vi "svl_Check Data Valid [Level] [Resampled] (N Ch).vi"(0 "scaled even angle signals [EU]":T5(array[cluster]) {"even angle signal" format="%.2f"; "dr" format="%.2f"; "r0" format="%.2f"}, 1 "exponential mode":enum16{"Slow", "Fast", "Impulse", "Custom"}(ring)=enum."Fast", 2 "time constant [ms]":dbl=125.0 format="%.2f", 5 "even angle channel info":T1[](array[typedef]) {"channel info"."pregain" format="%.2f"; "channel info"."weighting filter" items=["Linear", "A-weighting", "B-weighting", "C-weighting", "ITU-R 468-4", "Dolby", "CCITT", "C-message", "Wb", "Wc", "Wd", "We", "Wf", "Wh", "Wj", "Wk", "Wm", "AES17 20 kHz lowpass", "AES17 40 kHz lowpass", "AES17 20 kHz highpass", "AES17 40 kHz highpass"]; "channel info"."dB reference" format="%^.1e"; "channel info"."engineering units" items=["custom..."=0, "V"=1, "A"=21, "C"=30, "pC"=31, "s"=32, "-"=29, "Pa"=2, "N"=20, "g"=3, "m/s^2"=4, "m/s"=5, "m"=6, "mm/s"=12, "mm"=13, "micron/s"=14, "micron"=15, "in/s^2"=7, "in/s"=8, "in"=9, "mil/s"=10, "mil"=11, "rad/s^2"=16, "rad/s"=17, "rad"=18, "deg/s^2"=26, "deg/s"=27, "deg"=28, "RPM"=22, "cycle/s^2"=23, "Hz"=24, "cycle"=25, "strain"=19]; "channel info"."sensor sensitivity" format="%#_5f"}, 7 "level analysis":T7(ring), 9 "restart averaging (F)":bool, 11 "error in (no error)":errorcluster, 12 "integration time [s]":dbl=1.0 format="%.2f", 13 "decimation factor":i32=1 min=1 step=1) -> (4 "dup scaled even angle signals [EU]":T5(array[cluster]) {"even angle signal" format="%.2f"; "dr" format="%.2f"; "r0" format="%.2f"}, 6 "dup even angle channel info":T1[](array[typedef]) {"channel info"."pregain" format="%.2f"; "channel info"."weighting filter" items=["Linear", "A-weighting", "B-weighting", "C-weighting", "ITU-R 468-4", "Dolby", "CCITT", "C-message", "Wb", "Wc", "Wd", "We", "Wf", "Wh", "Wj", "Wk", "Wm", "AES17 20 kHz lowpass", "AES17 40 kHz lowpass", "AES17 20 kHz highpass", "AES17 40 kHz highpass"]; "channel info"."dB reference" format="%^.1e"; "channel info"."engineering units" items=["custom..."=0, "V"=1, "A"=21, "C"=30, "pC"=31, "s"=32, "-"=29, "Pa"=2, "N"=20, "g"=3, "m/s^2"=4, "m/s"=5, "m"=6, "mm/s"=12, "mm"=13, "micron/s"=14, "micron"=15, "in/s^2"=7, "in/s"=8, "in"=9, "mil/s"=10, "mil"=11, "rad/s^2"=16, "rad/s"=17, "rad"=18, "deg/s^2"=26, "deg/s"=27, "deg"=28, "RPM"=22, "cycle/s^2"=23, "Hz"=24, "cycle"=25, "strain"=19]; "channel info"."sensor sensitivity" format="%#_5f"}, 10 "processing state":T6(ring), 15 "error out":errorcluster)   [LabVIEW 2017]
uses:
  <vilib>/addons/_NISVFA/_Shared subVIs/Controls/svc_Resampled Channel Info.ctl
  <vilib>/addons/_NISVFA/_Shared subVIs/Controls/svc_Channel Info.ctl
  <vilib>/addons/_NISVFA/_Shared subVIs/Controls/svc_Engineering Units Text Ring.ctl
  <vilib>/addons/_NISVFA/_Shared subVIs/Controls/svc_Weighting Filter Text Ring.ctl
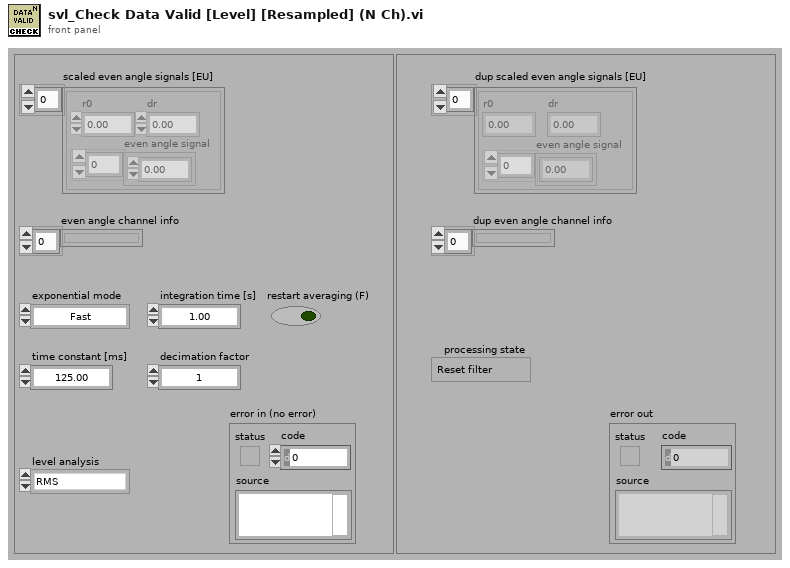
[diagram p1: front panel]
types:
  T1 = typedef "svc_Resampled Channel Info.ctl" = cluster{"channel name":string, "description":string, " channel info":T2}
  T2 = typedef "svc_Channel Info.ctl" = cluster{"sensor sensitivity":dbl, "engineering units":T3, "dB reference":dbl, "custom label":string, "weighting filter":T4, "pregain":dbl}
  T3 = typedef "svc_Engineering Units Text Ring.ctl" = u16
  T4 = typedef "svc_Weighting Filter Text Ring.ctl" = u16
  T5 = cluster{"r0":dbl, "dr":dbl, "even angle signal":dbl[]}[]
  T6 = enum16{"Reset filter", "Restart averaging", "Continue processing"}
  T7 = enum16{"RMS", "Running RMS", "Exp avg  ", "Dec exp avg ", "Peak", "Crest"}
  T8 = cluster{"ignore dt's equal":bool, "ignore array lengths equal":bool, "ignore # channels":bool}
  T9 = cluster{"ignore dt":bool, "ignore t0 continuity":bool, "ignore array length":bool, "ignore channel info":bool, "ignore channel name":bool}
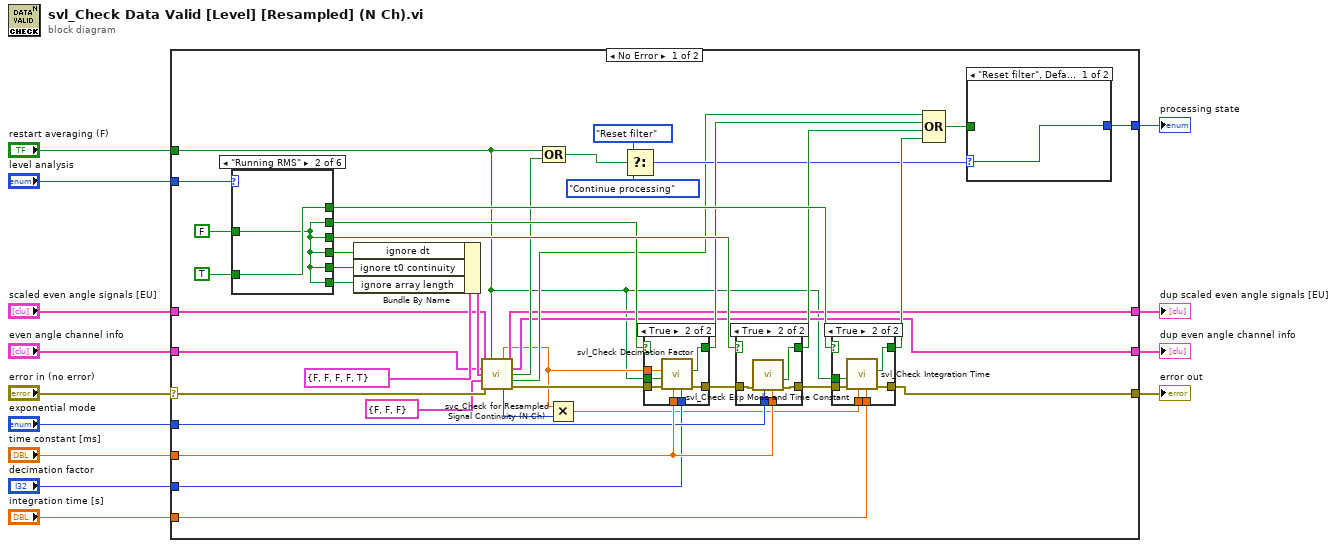
[diagram p0: block diagram]
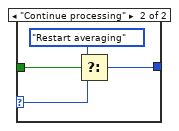
[diagram p10: hidden frame]
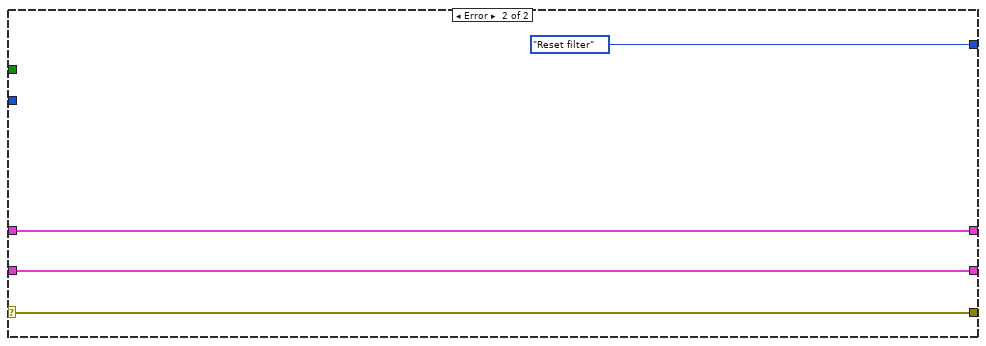
[diagram p11: hidden frame]
diagram:
  n1 = case shown="No Error" "error in (no error)" {
    selector: "error in (no error)" -> [w27 w98]
    tunnel: [w26 w98] -> w12
    tunnel: "scaled even angle signals [EU]" -> [w32 w96]
    tunnel: "restart averaging (F)" -> [w14 _]
    tunnel: "time constant [ms]" -> [w31 _]
    tunnel: [w53 T6."Reset filter" ("processing state")] -> w9
    tunnel: "level analysis" -> [w33 _]
    tunnel: "integration time [s]" -> [w28 _]
    tunnel: "decimation factor" -> [w29 _]
    tunnel: "exponential mode" -> [w30 _]
    tunnel: [w20 w96] -> w3
    tunnel: "even angle channel info" -> [w19 w95]
    tunnel: [w18 w95] -> w1
    frame No Error {
      n2 = case shown="\"Running RMS\"" w33 {
        tunnel: [w79 w80 w82 w84 w87 w89] -> w49
        tunnel: [w79 w80 w83 w84 w87 w89] -> w48
        tunnel: [w79 w81 w83 w85 w87 w89] -> w47
        tunnel: [w78 w80 w82 w84 w86 w88] -> w34
        tunnel: [w78 w80 w83 w85 w86 w88] -> w43
        tunnel: [w79 w80 w83 w85 w86 w89] -> w42
        tunnel: FALSE -> [w79 w80 w83 w85 w87 w89]
        tunnel: TRUE -> [w78 w81 w82 w84 w86 w88]
        frame "RMS", Default {
        }
        frame "Running RMS" {
        }
        frame "Exp avg  " {
        }
        frame "Dec exp avg " {
        }
        frame "Peak" {
        }
        frame "Crest" {
        }
      }
      n3 = Bundle By Name(cluster=T9 {"ignore dt"=FALSE, "ignore t0 continuity"=FALSE, "ignore array length"=FALSE, "ignore channel info"=FALSE, "ignore channel name"=TRUE} ("parameter controls"), "ignore dt"=w42, "ignore t0 continuity"=w43, "ignore array length"=w34) -> (w44:T9)
      n4 = call <vilib>:"svc_Check for Resampled Signal Continuity (N Ch).vi"("even angle signals"=w32, "restart averaging (F)"=w14, "even angle channel info"=w19, "parameter controls"=w44, "multichannel parameter controls"=T8 {"ignore dt's equal"=FALSE, "ignore array lengths equal"=FALSE, "ignore # channels"=FALSE}, "error in (no error)"=w27) -> ("dr"=w17:dbl, "dup even angle signals"=w20:T5, "dup even angle channel info"=w18:T1[], "waveform parameter changed"=w22:bool, "multichannel parameter changed"=w21:bool, "array length"=w16:i32, "error out"=w39:errorcluster)  [unwired: 3 in]
      n5 = Compound Arithmetic op=OR(w14, w22) -> (w46:bool)
      n6 = Multiply(x=w17, y=w16) -> (x*y=w15:dbl)
      n7 = Select(t=T6."Reset filter" ("processing state"), s=w46, f=T6."Continue processing" ("processing state")) -> (s? t:f=w25:T6)
      n8 = case shown="True" w48 {
        selector: w48 -> [w62 _]
        tunnel: w39 -> [w63 w70]
        tunnel: [w63 w69] -> w41
        tunnel: w31 -> [_ w68]
        tunnel: w29 -> [_ w67]
        tunnel: [w62 w65] -> w37
        tunnel: w17 -> [_ w66]
        tunnel: w14 -> [_ w64]
        frame False {
        }
        frame True {
          n9 = call <vilib>:"svl_Check Decimation Factor.vi"("decimation factor"=w67, "time constant [ms]"=w68, "error in (no error)"=w70, "restart averaging (F)"=w64, "dt"=w66) -> ("error out"=w69:errorcluster, "parameter has changed"=w65:bool)  [unwired: 5 in]
        }
      }
      n10 = case shown="True" w49 {
        selector: w49 -> [w71 _]
        tunnel: w30 -> [_ w77]
        tunnel: w41 -> [w72 w73]
        tunnel: [w72 w76] -> w40
        tunnel: [w71 w74] -> w38
        tunnel: w31 -> [_ w75]
        frame False {
        }
        frame True {
          n11 = call <vilib>:"svl_Check Exp Mode and Time Constant.vi"("time constant [ms]"=w75, "exponential mode"=w77, "error in (no error)"=w73) -> ("error out"=w76:errorcluster, "parameter has changed"=w74:bool)  [unwired: 7 in]
        }
      }
      n12 = case shown="True" w47 {
        selector: w47 -> [w54 _]
        tunnel: w40 -> [w55 w61]
        tunnel: [w55 w60] -> w26
        tunnel: w28 -> [_ w58]
        tunnel: [w54 w59] -> w52
        tunnel: w15 -> [_ w57]
        tunnel: w14 -> [_ w56]
        frame False {
        }
        frame True {
          n13 = call <vilib>:"svl_Check Integration Time.vi"("integration time"=w58, "acquisition period"=w57, "error in (no error)"=w61, "restart averaging (F)"=w56) -> ("error out"=w60:errorcluster, "parameter has changed"=w59:bool)  [unwired: 5 in, 1 out]
        }
      }
      n14 = Compound Arithmetic op=OR(w21, w37, w38, w52) -> (w24:bool)
      n15 = case shown="\"Reset filter\", Default" w25 {
        selector: w25 -> [w90 w93]
        tunnel: w24 -> [_ w94]
        tunnel: [w90 w91] -> w53
        frame "Reset filter", Default {
        }
        frame "Continue processing" {
          n16 = Select(t=T6."Restart averaging" ("processing state"), s=w94, f=w93) -> (s? t:f=w91:T6)
        }
      }
    }
    frame Error {
      (unwired) TRUE ("t0 changed")
    }
  }
  "error out" <- w12
  "processing state" <- w9
  "dup scaled even angle signals [EU]" <- w3
  "dup even angle channel info" <- w1
